vi "MakePath.vi"(0 "File Prefix":string="s", 1 "Root Data Folder":path=path "C:/Data", 2 "Index file":string="index.txt", 3 "Re-use index":i32=-1, 5 "Interactive":bool=TRUE, 7 "File middle":string, 9 "Extentions":string[](array[string])=[".tdms", ".txt", ".tdms_index"], 11 "Error In":errorcluster, 12 "Time Stamp (default 0 = now)":timestamp, 13 "Include time":bool, 14 "Index digits":i32=3) -> (4 "Paths out":path[](array[path]), 6 "format string":string="%03d", 8 "Try count":i32, 10 "Index out":i32=-1, 15 "Error Out":errorcluster)   [LabVIEW 2024]
panel:
  in  "Dashes?":bool
  in  "Split by day":bool=TRUE
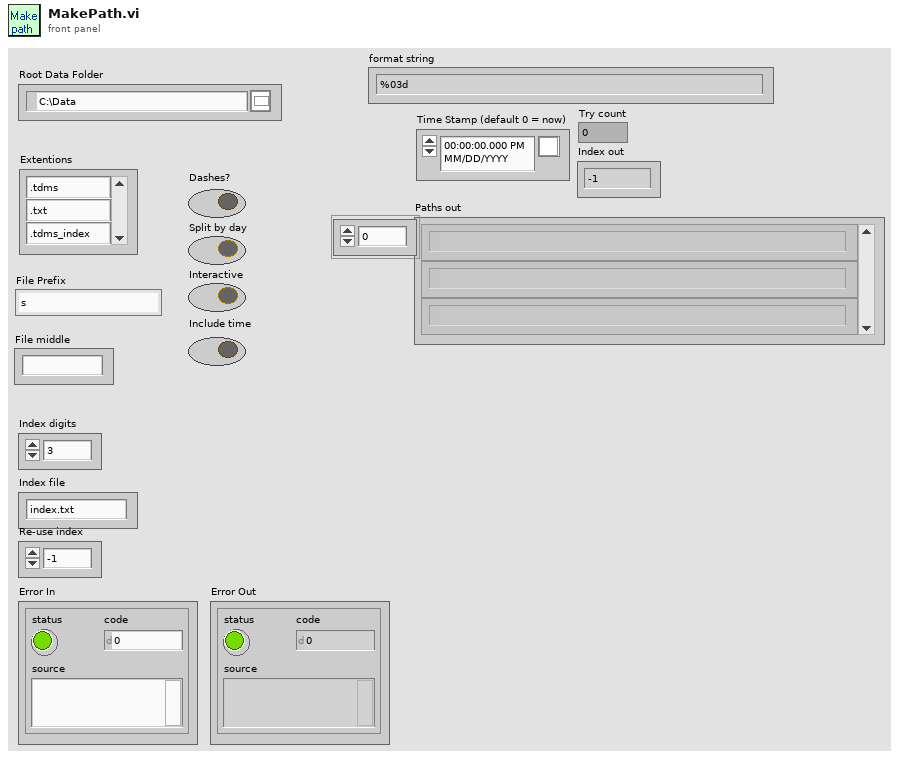
[diagram p1: front panel]
types:
  T1 = enum32{"existing file", "new file", "new or existing file", "existing dir", "new dir", "new or existing dir", "existing file (use LLBs)", "new file (use LLBs)", "new or existing file (use LLBs)", "new or existing file or directory (use LLBs)", "existing dir (use LLBs)", "new dir (use LLBs)", "new or existing dir (use LLBs)", "existing file or dir", "new file or dir", "new or existing file or dir", "existing file or dir (use LLBs)", "new file or dir (use LLBs)"}
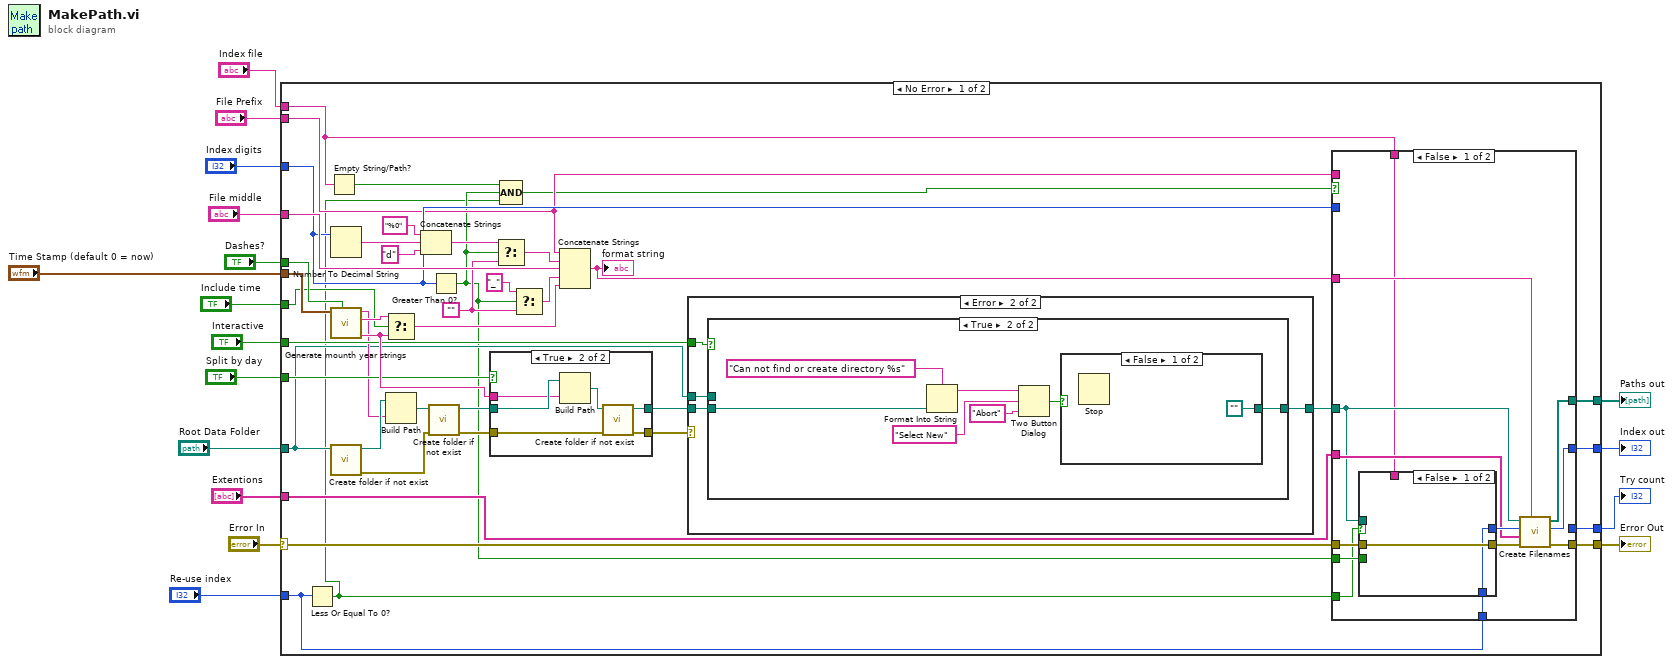
[diagram p0: block diagram]
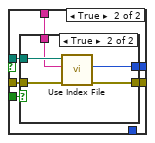
[diagram p3: hidden frame]
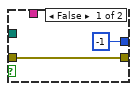
[diagram p4: hidden frame]
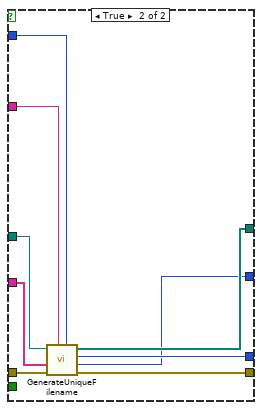
[diagram p5: hidden frame]
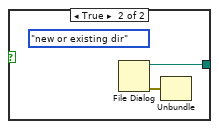
[diagram p8: hidden frame]
diagram:
  n1 = case shown="No Error" "Error In" {
    selector: "Error In" -> [w35 w121]
    tunnel: [w55 w121] -> w16
    tunnel: "Index digits" -> [w31 _]
    tunnel: "Time Stamp (default 0 = now)" -> [w49 _]
    tunnel: "Root Data Folder" -> [w41 _]
    tunnel: "Dashes?" -> [w48 _]
    tunnel: "Split by day" -> [w47 _]
    tunnel: "Interactive" -> [w46 _]
    tunnel: "Include time" -> [w45 _]
    tunnel: "File Prefix" -> [w30 _]
    tunnel: "Extentions" -> [w40 _]
    tunnel: "File middle" -> [w39 _]
    tunnel: [w38 _] -> w5
    tunnel: [w37 _] -> w4
    tunnel: "Index file" -> [w20 _]
    tunnel: [w21 _] -> w2
    tunnel: "Re-use index" -> [w18 _]
    frame No Error {
      w25 = ""
      n2 = Less Or Equal To 0?(x=w18) -> (x <= 0?=w19:bool)
      n3 = Empty String/Path?(string/path=w20) -> (empty?=w29:bool)
      n4 = Number To Decimal String(number=w31) -> (decimal integer string=w33:string)  [unwired: 1 in]
      n5 = call "Generate mounth year strings.vi"("Dashes?"=w48, "Time Stamp (default 0 = now)"=w49) -> ("mmdd"=w51:string, "hhmmss_mmdd"=w52:string, "Month_year"=w43:string)  [unwired: 7 out]
      n6 = call "Create folder if not exist.vi"("Folder Path Control"=w41) -> ("Error Out"=w59:errorcluster, "Folder Path out"=w44:path)  [unwired: 1 in, 8 out]
      n7 = Select(t=w52, s=w45, f=w51) -> (s? t:f=w50:string)
      n8 = Build Path(base path=w44, name or relative path=w43) -> (appended path=w42:path)
      n9 = Concatenate Strings("%0" ("Substring"), w33, "d" ("Substring")) -> (w28:string)
      n10 = call "Create folder if not exist.vi"("Error In"=w59, "Folder Path Control"=w42) -> ("Error Out"=w57:errorcluster, "Folder Path out"=w58:path)  [unwired: 8 out]
      n11 = Greater Than 0?(x=w31) -> (x > 0?=w22:bool)
      n12 = case shown="True" w47 {
        tunnel: w58 -> [w60 w64]
        tunnel: w57 -> [w61 w67]
        tunnel: [w60 w66] -> w56
        tunnel: [w61 w65] -> w54
        tunnel: w51 -> [_ w63]
        frame False {
        }
        frame True {
          n13 = Build Path(base path=w64, name or relative path=w63) -> (appended path=w62:path)
          n14 = call "Create folder if not exist.vi"("Error In"=w67, "Folder Path Control"=w62) -> ("Error Out"=w65:errorcluster, "Folder Path out"=w66:path)  [unwired: 8 out]
        }
      }
      n15 = Select(t=w28, s=w22, f=w25) -> (s? t:f=w27:string)
      n16 = Compound Arithmetic op=AND(w29, w22, w19) -> (w23:bool)
      n17 = Select(t="_" ("string"), s=w22, f=w25) -> (s? t:f=w24:string)
      n18 = Concatenate Strings(w30, w27, w39, w24, w50) -> (w53:string)
      "format string" <- w53
      n19 = case shown="Error" w54 {
        tunnel: w56 -> [w105 w107]
        tunnel: w46 -> [_ w109]
        tunnel: [w105 w108] -> w36
        tunnel: w41 -> [_ w106]
        frame No Error {
        }
        frame Error {
          n20 = case shown="True" w109 {
            tunnel: [w110 w111] -> w108
            tunnel: w107 -> [_ w115]
            tunnel: w106 -> [w110 _]
            frame False {
            }
            frame True {
              n21 = Format Into String(format string="Can not find or create directory %s" ("Format String"), w115) -> (resulting string=w113:string)  [unwired: 2 in, 1 out]
              n22 = Two Button Dialog(message=w113, 1:"Abort" ("F button name (\"Cancel\")"), 2:"Select New" ("T button name (\"OK\")")) -> (T button?=w112:bool)
              n23 = case shown="False" w112 {
                tunnel: [path "" w120] -> w111
                frame False {
                  n24 = Stop() -> ()  [unwired: 1 out]
                }
                frame True {
                  (unwired) T1."new or existing dir" ("select mode (2)")
                  n25 = File Dialog() -> (0:w119:errorcluster, 3:w120:path)  [unwired: 1 in, 8 out]
                  n26 = Unbundle(w119) -> ()  [unwired: 3 out]
                }
              }
            }
          }
        }
      }
      n27 = case shown="False" w23 {
        tunnel: [w79 w102] -> w37
        tunnel: w36 -> [w73 w98]
        tunnel: w30 -> [_ _]
        tunnel: [w80 w104] -> w55
        tunnel: w40 -> [w74 w103]
        tunnel: w53 -> [w75 w101]
        tunnel: w35 -> [w78 w100]
        tunnel: w31 -> [_ w99]
        tunnel: [_ w97] -> w38
        tunnel: w22 -> [w72 _]
        tunnel: [w71 w96] -> w21
        tunnel: w20 -> [w70 _]
        tunnel: w19 -> [w69 _]
        tunnel: w18 -> [w68 _]
        frame False {
          n28 = case shown="False" w69 {
            tunnel: w78 -> [w82 w88]
            tunnel: [w82 w87] -> w77
            tunnel: [w81 w86] -> w76
            tunnel: w73 -> [_ w85]
            tunnel: w72 -> [_ w84]
            tunnel: w70 -> [_ w83]
            tunnel: w68 -> [w81 _]
            frame False {
            }
            frame True {
              n29 = case shown="True" w84 {
                tunnel: w88 -> [w90 w95]
                tunnel: [w90 w94] -> w87
                tunnel: [-1 ("Index") w93] -> w86
                tunnel: w85 -> [_ w92]
                tunnel: w83 -> [_ w91]
                frame False {
                }
                frame True {
                  n30 = call "Use Index File.vi"("error in"=w95, "Index file"=w91, "Folder Path"=w92) -> ("error out"=w94:errorcluster, "Index"=w93:i32)  [unwired: 7 in]
                }
              }
            }
          }
          n31 = call "Create Filenames.vi"("Format string"=w75, "Error In"=w77, "File name suffixes"=w74, "Index"=w76, "Folder Path Control"=w73) -> ("Error Out"=w80:errorcluster, "Index out"=w71:i32, "Paths"=w79:path[])  [unwired: 4 in]
        }
        frame True {
          n32 = call "GenerateUniqueFilename.vi"("Index digits"=w99, "format string"=w101, "Error In"=w100, "File name suffixes"=w103, "Folder Path Control"=w98) -> ("Error Out"=w104:errorcluster, "Index out"=w96:i32, "Try count"=w97:i32, "Paths"=w102:path[])  [unwired: 3 out]
        }
      }
    }
    frame Error {
    }
  }
  "Error Out" <- w16
  "Try count" <- w5
  "Paths out" <- w4
  "Index out" <- w2
